vi "ThreadUI.vi"(4 "数据通知器":refnum<notifier>, 5 "Angle Data Queue":refnum<queue> caption="角度数据队列", 6 "User Event - Stop":refnum<user-event> caption="用户事件－停止", 7 "Analog Data Queue":refnum<queue> caption="模拟数据队列", 8 "error in (no error)":errorcluster caption="错误输入（无错误）", 10 "Measurement UI Controls":T1 caption="测量UI控件", 11 "Message Queues":T2 caption="消息队列") -> (0 "error out":errorcluster caption="错误输出")   [LabVIEW 2015]
uses:
  support/Message Queue/All Message Queues.ctl
  support/Message Queue/Message Cluster.ctl
  controls/UI Data.ctl
  Settings/Settings.ctl
  Acquisition/Hardware Configuration.ctl
  Logging/Logging Configuration.ctl
  Action/Hardware Configuration.ctl
  TaskMan/TaskMan Configuration.ctl
  TaskMan/TaskSettings.ctl
  controls/UI State.ctl
  Measure Type.ctl
  <vilib>/Analysis/baseanly.llb/Mean (DBL).vi
  support/Message Queue/Enqueue Message (Single).vi
  <vilib>/Utility/xml.llb/Write to XML File(string).vi
  <vilib>/Utility/error.llb/Error Cluster From Error Code.vi
  <vilib>/ErrorRing/Error Ring.xnode
  support/Message Queue/Message Queue.lvlib
  Acquisition/Acquisition.lvlib
  Logging/Logging.lvlib
  Action/Action.lvlib
  Settings/Settings.lvlib
  TaskMan/TaskMan.lvlib
  support/User Event - Stop/User Event - Stop.lvlib
  <vilib>/Analysis/NI_AALBase.lvlib
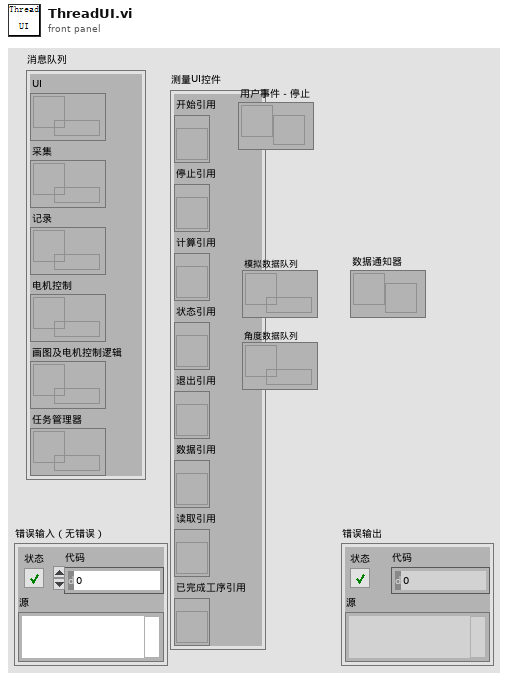
[diagram p1: front panel]
types:
  T1 = typedef "UI Data.ctl" = cluster{"Start Ref":refnum<vi>, "Stop Ref":refnum<vi>, "calculate Ref":refnum<vi>, "Status Ref":refnum<vi>, "Exit Ref":refnum<vi>, "read Ref":refnum<vi>, "clean Ref":refnum<vi>, "Finish Ref":refnum<vi>}
  T2 = typedef "Message Queue.lvlib/All Message Queues.ctl" = cluster{"UI":refnum<queue>, "Acquisition":refnum<queue>, "Logging":refnum<queue>, "plot logic":refnum<queue>, "Action Control":refnum<queue>, "TaskMan":refnum<queue>}
  T3 = typedef "UI State.ctl" = enum16{"Idle", "Acquiring and Logging", "Waiting for Exit", "Waiting for Exit (Acq Stopped)", "Waiting for Exit (Log Stopped)", "Waiting for Stop", "Waiting for Stop (Acq Stopped)", "Waiting for Stop (Log Stopped)"}
  T4 = typedef "Settings.lvlib/Settings.ctl" = cluster{"Hardware Configuration":T5, "Logging Configuration":T6, "Action Configuration":T7, "所有测试项目任务":T18}
  T5 = typedef "Acquisition.lvlib/Hardware Configuration.ctl" = cluster{"电压读取设置":cluster{"DAQmx Channel":tag, "Max Input":dbl, "Min Input":dbl, "Sample Rate":dbl, "Sample Number":i32, "DAQmx Task":refnum<k21>, "device in":tag}, "角度传感器设置":cluster{"counter":tag, "units":i32, "分辨率":i32, "初始角度":dbl, "DecodingType":i32, "A相端口":tag, "B相端口":tag, "task in":refnum<k21>}}
  T6 = typedef "Logging.lvlib/Logging Configuration.ctl" = cluster{"Log File Base Path":path, "电压传感器转换率":dbl[], "电压传感器本底":dbl[], "测试模式是否需要保存数据？":bool}
  T7 = typedef "Action.lvlib/Hardware Configuration.ctl" = cluster{"PLC设置":T8, "动作设置":T9, "电机设置":T13, "所有测试电机转动逻辑":T14}
  T8 = typedef "Action.lvlib/PLC设置.ctl" = cluster{"ActLogicalStationNumber":i32, "ActUtlType":refnum<k7>}
  T9 = typedef "Action.lvlib/动作设置.ctl" = cluster{"自动跳法测试动作":T10, "其他动作":T12}
  T10 = typedef "Action.lvlib/自动调阀测试动作设置.ctl" = cluster{"夹紧阀总":T11, "夹紧/松阀芯":T11, "方向机供油":T11, "扭杆紧/松":T11, "电机使能":T11, "内泄漏开":T11, "内泄漏停":T11, "数控钻孔启动":T11, "托起缸上":T11, "托起缸下":T11, "内泄漏放油":T11, "读取开始按钮":T11, "读取压销启动":T11, "读取压销完成":T11, "放松阀总":T11, "卡盘松紧":T11}
  T11 = typedef "Action.lvlib/PLC控制指令.ctl" = cluster{"变量类型":u32, "PLC地址":i32, "size":i32, "写入数据(写入时有效)":i16}
  T12 = typedef "Action.lvlib/其他动作设置 .ctl" = cluster{"其他指令1":T11, "其他指令2":T11, "其他指令3":T11, "其他指令4":T11, "其他指令5":T11}
  T13 = typedef "Action.lvlib/电机控制设置.ctl" = cluster{"counter":tag, "方向端口":tag, "当前方向":bool, "频率":dbl, "DAQmx Task":refnum<k21>, "一圈脉冲数":i32}
  T14 = typedef "Action.lvlib/所有测试电机转动逻辑.ctl" = cluster{"啮合测试电机转动逻辑":T15, "退回测试电机转动逻辑":T15, "功能测试电机转动逻辑":T15, "力特性测试电机转动逻辑":T15, "自动调阀测试分中电机转动逻辑":T15, "自动调阀测试对中电机转动逻辑":T15, "内泄漏电机转动逻辑":T15}
  T15 = typedef "Action.lvlib/电机转动逻辑1.ctl" = cluster{"反转判断条件1":T16, "停止判断条件1":T17}
  T16 = typedef "Action.lvlib/反转判断条件1.ctl" = cluster{"传感器序号":i32, "条件":enum16{"小于", "大于", "等于"}, "值":dbl, "条件判断时间间隔":i32}
  T17 = typedef "Action.lvlib/停止判断条件1.ctl" = cluster{"传感器序号":i32, "正转/反转":enum16{"正转", "反转"}, "反转次数":i32, "停止角度":dbl, "停止误差范围":dbl}
  T18 = typedef "TaskMan.lvlib/TaskMan Configuration.ctl" = cluster{"全自动调阀任务列表":T19}
  T19 = typedef "TaskMan.lvlib/全自动调阀任务列表.ctl" = T20[]
  T20 = typedef "TaskMan.lvlib/TaskSettings.ctl" = cluster{"任务指令":string, "等待时间":dbl}
  T21 = typedef "Measure Type.ctl" = enum16{"啮合", "退回", "功能", "力特性", "内泄漏", "分中", "对中"}
  T22 = enum8{"Enabled", "Disabled", "Disabled and Grayed Out"}
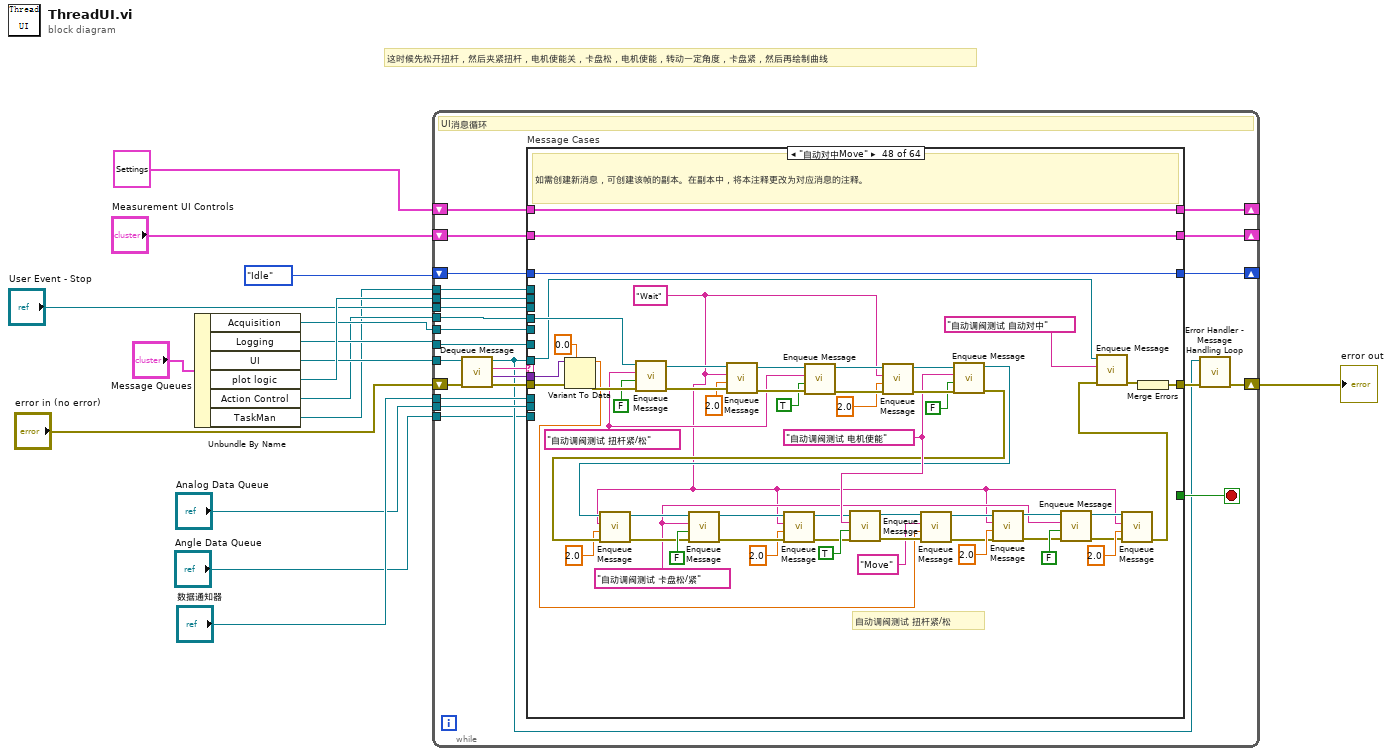
[diagram p0: block diagram]
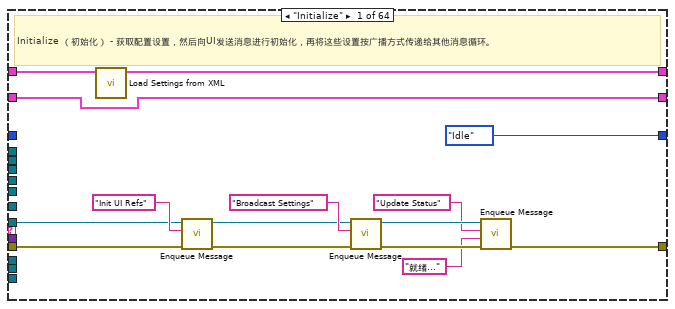
[diagram p2: hidden frame]
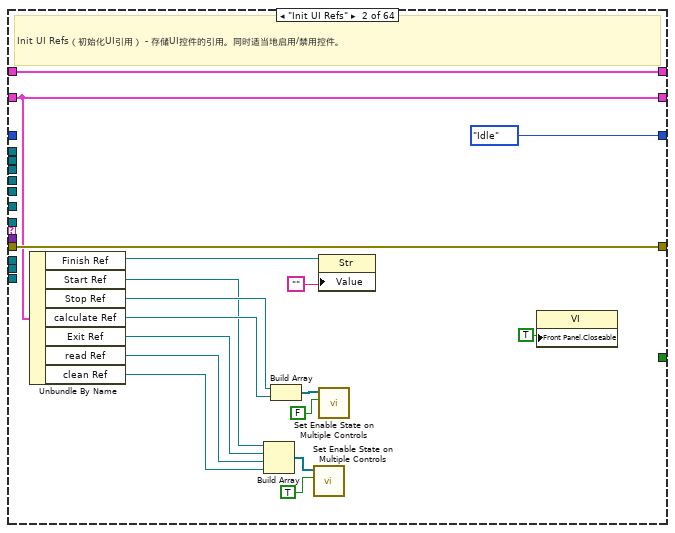
[diagram p3: hidden frame]
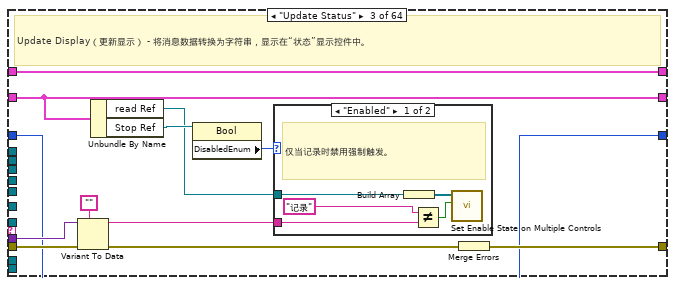
[diagram p4: hidden frame]
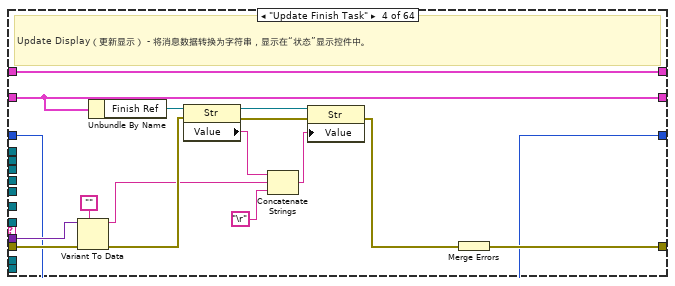
[diagram p6: hidden frame]
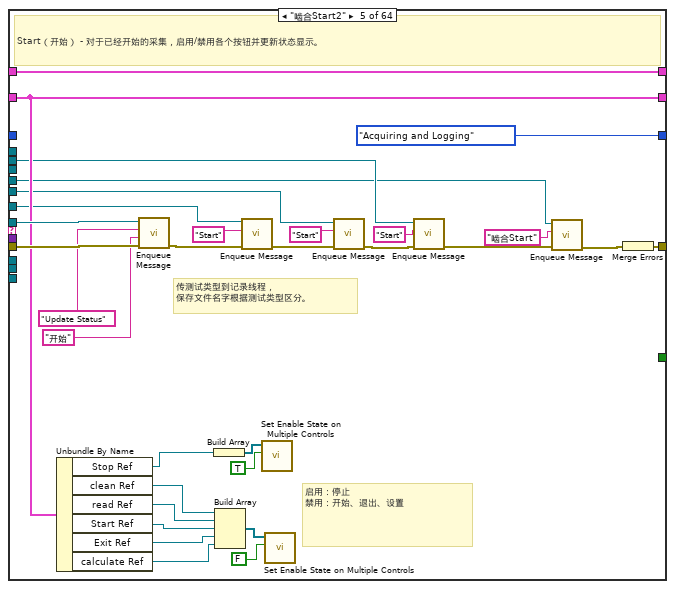
[diagram p7: hidden frame]
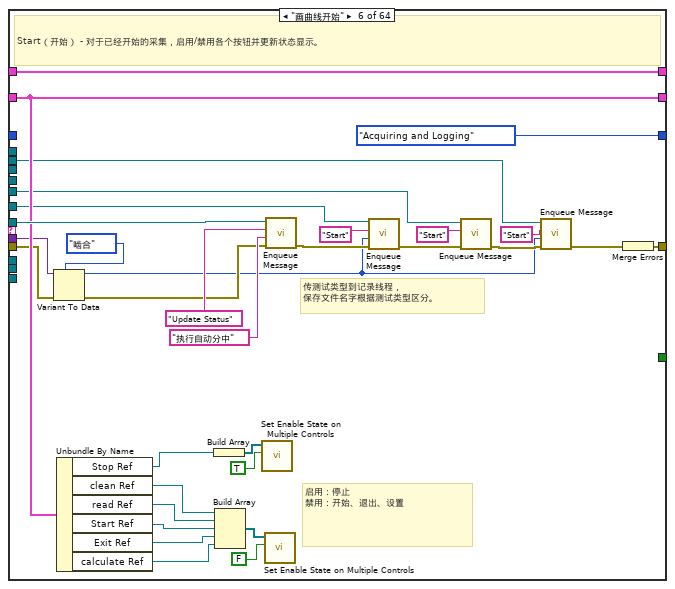
[diagram p8: hidden frame]
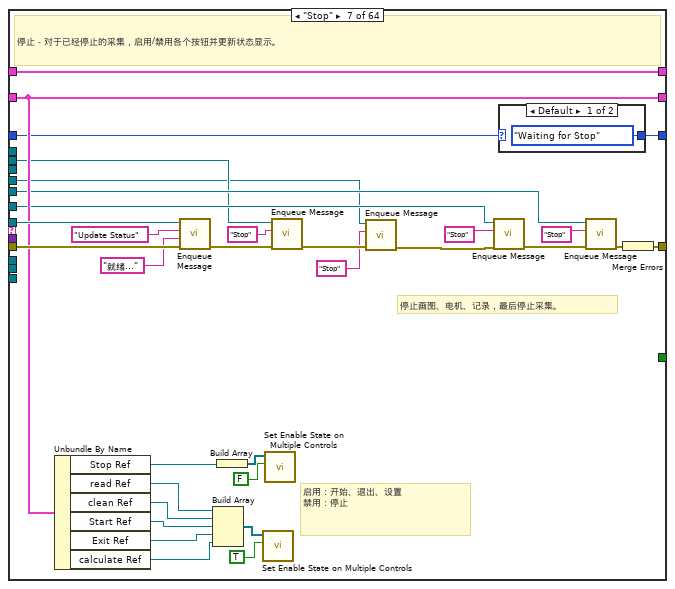
[diagram p9: hidden frame]
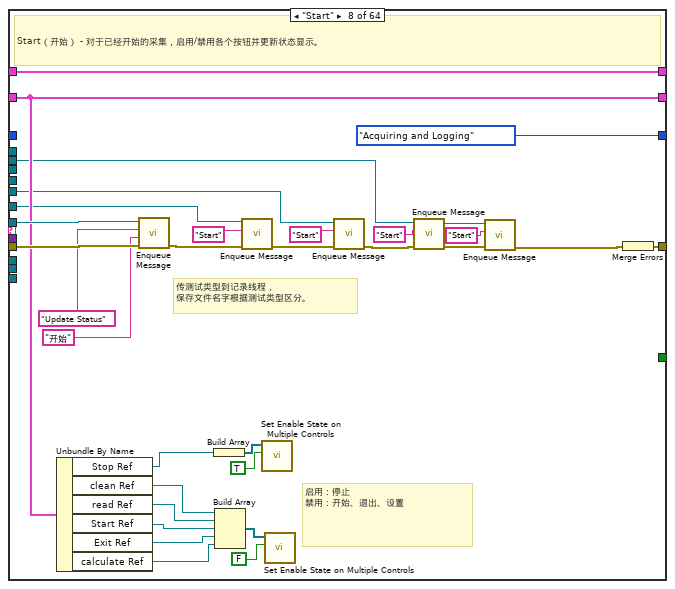
[diagram p11: hidden frame]
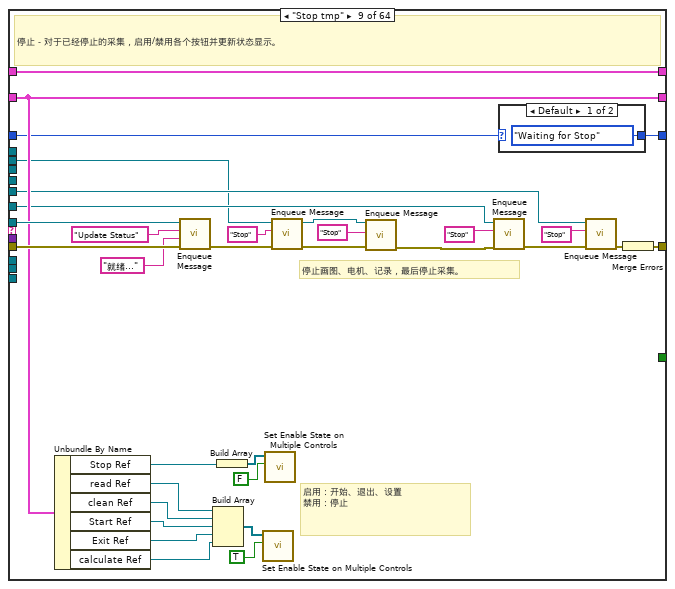
[diagram p12: hidden frame]
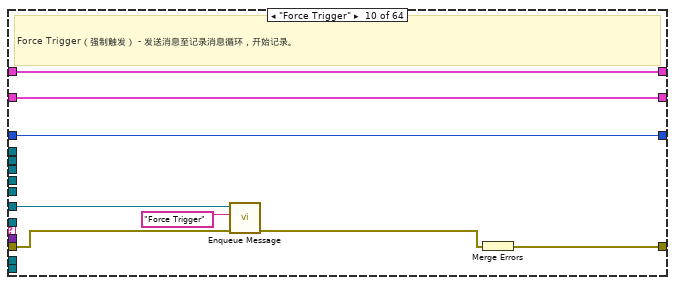
[diagram p14: hidden frame]
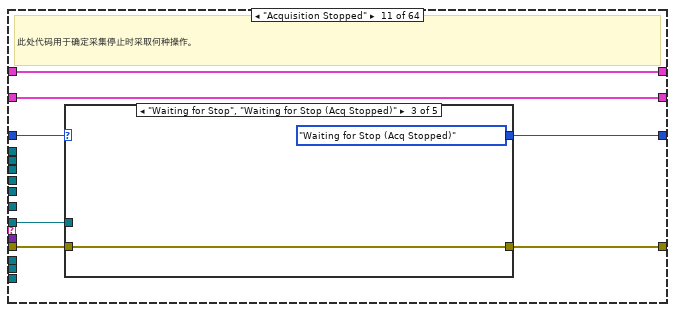
[diagram p15: hidden frame]
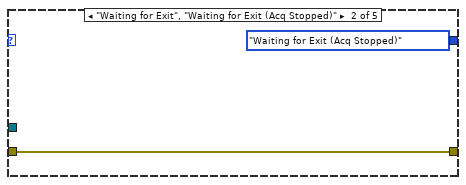
[diagram p17: hidden frame]
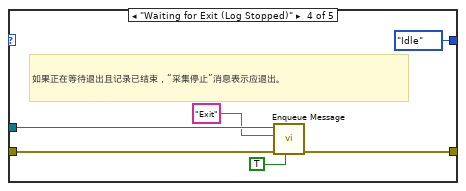
[diagram p18: hidden frame]
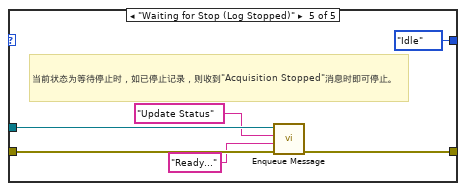
[diagram p19: hidden frame]
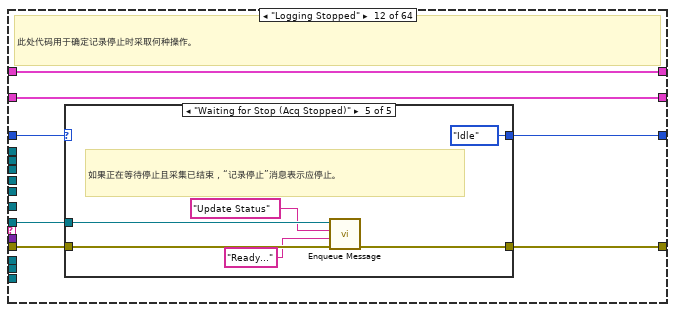
[diagram p20: hidden frame]
diagram:
  # "这时候先松开扭杆，然后夹紧扭杆，电机使能关，卡盘松，电机使能，转动一定角度，卡盘紧，然后再绘制曲线"
  n1 = Unbundle By Name("Message Queues") -> ("Acquisition"=w12:refnum<queue>, "Logging"=w13:refnum<queue>, "UI"=w14:refnum<queue>, "plot logic"=w15:refnum<queue>, "Action Control"=w2:refnum<queue>, "TaskMan"=w1:refnum<queue>)
  n2 = while {
    tunnel: w14 -> [w34]
    tunnel: "User Event - Stop" -> [w39]
    shift-right: [w24] -> w4
    shift-left: "error in (no error)" -> [w38]
    shift-right: [w33] -> _
    shift-left: T4 {"Hardware Configuration"={"电压读取设置"={"DAQmx Channel"="", "Max Input"=0.0, "Min Input"=0.0, "Sample Rate"=0.0, "Sample Number"=0, "DAQmx Task"="", "device in"=""}, "角度传感器设置"={"counter"="Dev1/ctr0", "units"=10146, "分辨率"=0, "初始角度"=0.0, "DecodingType"=10092, "A相端口"="/Dev1/PFI8", "B相端口"="/Dev1/PFI8", "task in"=""}}, "Logging Configuration"={"Log File Base Path"=path "", "电压传感器转换率"=[], "电压传感器本底"=[], "测试模式是否需要保存数据？"=FALSE}, "Action Configuration"={"PLC设置"={"ActLogicalStationNumber"=9600, "ActUtlType"=refnum}, "动作设置"={"自动跳法测试动作"={"夹紧阀总"={"变量类型"=2, "PLC地址"=0, "size"=0, "写入数据(写入时有效)"=0}, "夹紧/松阀芯"={"变量类型"=2, "PLC地址"=0, "size"=0, "写入数据(写入时有效)"=0}, "方向机供油"={"变量类型"=2, "PLC地址"=0, "size"=0, "写入数据(写入时有效)"=0}, "扭杆紧/松"={"变量类型"=2, "PLC地址"=0, "size"=0, "写入数据(写入时有效)"=0}, "电机使能"={"变量类型"=2, "PLC地址"=0, "size"=0, "写入数据(写入时有效)"=0}, "内泄漏开"={"变量类型"=2, "PLC地址"=0, "size"=0, "写入数据(写入时有效)"=0}, "内泄漏停"={"变量类型"=2, "PLC地址"=0, "size"=0, "写入数据(写入时有效)"=0}, "数控钻孔启动"={"变量类型"=2, "PLC地址"=0, "size"=0, "写入数据(写入时有效)"=0}, "托起缸上"={"变量类型"=2, "PLC地址"=0, "size"=0, "写入数据(写入时有效)"=0}, "托起缸下"={"变量类型"=2, "PLC地址"=0, "size"=0, "写入数据(写入时有效)"=0}, "内泄漏放油"={"变量类型"=2, "PLC地址"=0, "size"=0, "写入数据(写入时有效)"=0}, "读取开始按钮"={"变量类型"=2, "PLC地址"=0, "size"=0, "写入数据(写入时有效)"=0}, "读取压销启动"={"变量类型"=2, "PLC地址"=0, "size"=0, "写入数据(写入时有效)"=0}, "读取压销完成"={"变量类型"=2, "PLC地址"=0, "size"=0, "写入数据(写入时有效)"=0}, "放松阀总"={"变量类型"=2, "PLC地址"=0, "size"=0, "写入数据(写入时有效)"=0}, "卡盘松紧"={"变量类型"=2, "PLC地址"=0, "size"=0, "写入数据(写入时有效)"=0}}, "其他动作"={"其他指令1"={"变量类型"=2, "PLC地址"=0, "size"=0, "写入数据(写入时有效)"=0}, "其他指令2"={"变量类型"=2, "PLC地址"=0, "size"=0, "写入数据(写入时有效)"=0}, "其他指令3"={"变量类型"=2, "PLC地址"=0, "size"=0, "写入数据(写入时有效)"=0}, "其他指令4"={"变量类型"=2, "PLC地址"=0, "size"=0, "写入数据(写入时有效)"=0}, "其他指令5"={"变量类型"=2, "PLC地址"=0, "size"=0, "写入数据(写入时有效)"=0}}}, "电机设置"={"counter"="Dev1/ctr0", "方向端口"="", "当前方向"=FALSE, "频率"=0.0, "DAQmx Task"="", "一圈脉冲数"=0}, "所有测试电机转动逻辑"={"啮合测试电机转动逻辑"={"反转判断条件1"={"传感器序号"=0, "条件"=enum."小于", "值"=0.0, "条件判断时间间隔"=0}, "停止判断条件1"={"传感器序号"=0, "正转/反转"=enum."正转", "反转次数"=0, "停止角度"=0.0, "停止误差范围"=0.0}}, "退回测试电机转动逻辑"={"反转判断条件1"={"传感器序号"=0, "条件"=enum."小于", "值"=0.0, "条件判断时间间隔"=0}, "停止判断条件1"={"传感器序号"=0, "正转/反转"=enum."正转", "反转次数"=0, "停止角度"=0.0, "停止误差范围"=0.0}}, "功能测试电机转动逻辑"={"反转判断条件1"={"传感器序号"=0, "条件"=enum."小于", "值"=0.0, "条件判断时间间隔"=0}, "停止判断条件1"={"传感器序号"=0, "正转/反转"=enum."正转", "反转次数"=0, "停止角度"=0.0, "停止误差范围"=0.0}}, "力特性测试电机转动逻辑"={"反转判断条件1"={"传感器序号"=0, "条件"=enum."小于", "值"=0.0, "条件判断时间间隔"=0}, "停止判断条件1"={"传感器序号"=0, "正转/反转"=enum."正转", "反转次数"=0, "停止角度"=0.0, "停止误差范围"=0.0}}, "自动调阀测试分中电机转动逻辑"={"反转判断条件1"={"传感器序号"=0, "条件"=enum."小于", "值"=0.0, "条件判断时间间隔"=0}, "停止判断条件1"={"传感器序号"=0, "正转/反转"=enum."正转", "反转次数"=0, "停止角度"=0.0, "停止误差范围"=0.0}}, "自动调阀测试对中电机转动逻辑"={"反转判断条件1"={"传感器序号"=0, "条件"=enum."小于", "值"=0.0, "条件判断时间间隔"=0}, "停止判断条件1"={"传感器序号"=0, "正转/反转"=enum."正转", "反转次数"=0, "停止角度"=0.0, "停止误差范围"=0.0}}, "内泄漏电机转动逻辑"={"反转判断条件1"={"传感器序号"=0, "条件"=enum."小于", "值"=0.0, "条件判断时间间隔"=0}, "停止判断条件1"={"传感器序号"=0, "正转/反转"=enum."正转", "反转次数"=0, "停止角度"=0.0, "停止误差范围"=0.0}}}}, "所有测试项目任务"={"全自动调阀任务列表"=[]}} ("Settings") -> [w32]
    shift-right: [w30] -> _
    shift-left: "Measurement UI Controls" -> [w31]
    tunnel: w12 -> [w29]
    tunnel: w13 -> [w28]
    tunnel: "数据通知器" -> [w27]
    tunnel: "Analog Data Queue" -> [w26]
    shift-right: [w21] -> _
    shift-left: UI_State."Idle" ("UI State") -> [w22]
    tunnel: w15 -> [w19]
    tunnel: "Angle Data Queue" -> [w20]
    tunnel: w2 -> [w18]
    tunnel: w1 -> [w17]
    stop <- w40 stop-if-true
    # "UI消息循环"
    n3 = call "Dequeue Message.vi"("error in (no error)"=w38, "Message Queue"=w34) -> ("error out"=w37:errorcluster, "Message Data"=w35:variant, "Message"=w36:string, "dup Message Queue"=w23:refnum<queue>)  [unwired: 6 in]
    n4 = case "Message Cases" shown="\"自动对中Move\"" w36 {
      selector: w36 -> [_ _ _ _ _ _ _ _ _ _ _ _ _ _ _ _ _ _ _ _ _ _ _ _ _ _ _ _ _ _ _ _ _ _ _ _ _ _ _ _ _ _ _ _ _ _ _ _ _ _ _ _ _ _ _ _ _ _ _ _ _ _ _ w946]
      tunnel: w23 -> [w45 _ _ _ w135 w167 w199 w232 w264 _ w276 w301 _ w350 w370 w376 w415 _ _ _ _ w475 w487 w499 w511 _ _ w537 _ _ _ _ _ _ _ w621 _ _ _ _ _ w686 _ _ w712 _ _ w740 w797 _ _ _ _ _ _ _ _ w880 w901 _ _ _ w934 _]
      tunnel: w37 -> [w44 w72 w83 w104 w134 w141 w198 w231 w263 w272 w278 w303 w333 w351 w363 w375 w422 w429 w436 w447 w460 w474 w486 w498 w510 w516 w526 w540 w552 w566 w574 w585 w594 w603 w612 w619 w636 w645 w653 w662 w671 w685 w694 w700 w710 w727 w735 w790 w799 w811 w819 w828 w836 w844 w853 w862 w871 w878 w900 w907 w916 w925 w932 _]
      tunnel: [w51 w72 w84 w105 w136 w168 w200 w233 w265 w275 w277 w302 w343 w348 w366 w374 w423 w428 w443 w452 w464 w476 w488 w500 w512 w519 w530 w543 w556 w569 w581 w589 w598 w607 w616 w631 w640 w649 w657 w666 w675 w687 w699 w707 w722 w731 w739 w794 w806 w815 w823 w832 w840 w848 w857 w866 w875 w890 w902 w911 w920 w929 w944 w947] -> w25
      tunnel: [_ _ _ _ _ _ _ _ _ _ _ _ _ _ _ _ TRUE _ _ _ _ _ _ _ _ _ _ _ _ _ _ _ _ _ _ _ _ _ _ _ _ _ _ _ _ _ _ _ _ _ _ _ _ _ _ _ _ _ _ _ _ _ _ _] -> w40
      tunnel: w35 -> [_ _ w82 w103 _ w140 _ _ _ _ _ _ _ _ w362 _ _ _ w434 w444 w459 _ _ _ _ _ _ _ _ _ w572 _ w590 w599 w608 _ w632 w641 _ w658 w667 _ w693 _ _ _ _ w789 _ w807 _ w824 _ _ _ _ _ _ _ _ _ _ _ _]
      tunnel: w39 -> [_ _ _ _ _ _ _ _ _ _ _ _ _ _ _ _ w421 _ _ _ _ _ _ _ _ _ _ _ _ _ _ _ _ _ _ _ _ _ _ _ _ _ _ _ _ _ _ _ _ _ _ _ _ _ _ _ _ _ _ _ _ _ _ _]
      tunnel: [w54 w71 w79 w101 w133 w166 w197 w230 w262 w274 w282 w307 w341 w349 w372 w379 w419 w427 w430 w451 w463 w473 w485 w497 w509 w514 w527 w533 w553 w564 w580 w588 w595 w604 w613 w630 w637 w646 w654 w663 w672 w684 w688 w702 w721 w728 w736 w793 w803 w812 w820 w829 w837 w847 w856 w865 w874 w889 w899 w910 w919 w928 w943 w949] -> w33
      tunnel: w32 -> [w55 w71 w79 w101 w133 w166 w197 w230 w262 w274 w282 w307 w341 w352 w372 w379 w419 w427 w432 w451 w463 w473 w485 w497 w509 w514 w527 w534 w553 w564 w580 w588 w595 w604 w613 w630 w637 w646 w654 w663 w672 w684 w688 w702 w721 w728 w736 w793 w803 w812 w820 w829 w837 w847 w856 w865 w874 w889 w899 w910 w919 w928 w943 w949]
      tunnel: w31 -> [w47 w58 w78 w100 w130 w163 w194 w227 w259 w273 w281 w306 w338 w347 w371 w378 w418 w426 w442 w450 w462 w471 w483 w495 w507 w518 w529 w542 w555 w568 w579 w587 w597 w606 w615 w628 w639 w648 w656 w665 w674 w682 w698 w706 w719 w730 w738 w792 w805 w814 w822 w831 w839 w846 w855 w864 w873 w887 w897 w909 w918 w927 w941 w948]
      tunnel: [w47 w58 w78 w100 w130 w163 w194 w227 w259 w273 w281 w306 w338 w347 w371 w378 w418 w426 w442 w450 w462 w471 w483 w495 w507 w518 w529 w542 w555 w568 w579 w587 w597 w606 w615 w628 w639 w648 w656 w665 w674 w682 w698 w706 w719 w730 w738 w792 w805 w814 w822 w831 w839 w846 w855 w864 w873 w887 w897 w909 w918 w927 w941 w948] -> w30
      tunnel: w29 -> [_ _ _ _ w118 w151 w182 w215 w247 _ _ _ w337 _ _ _ w417 _ _ _ _ _ _ _ _ _ w525 _ w551 _ _ _ _ _ _ _ _ _ _ _ _ _ _ _ _ _ _ _ _ _ _ _ _ _ _ _ _ _ _ _ _ _ _ _]
      tunnel: w28 -> [_ _ _ _ w120 w153 w185 w217 w250 w269 _ _ w336 _ _ _ w416 _ _ _ _ _ _ _ _ _ w522 _ w548 _ w576 w582 _ _ _ _ _ _ _ _ _ _ _ w701 _ w723 w732 _ _ _ _ _ _ _ _ _ _ _ _ _ _ _ _ _]
      tunnel: w27 -> [_ _ _ _ _ _ _ _ _ _ _ _ _ _ _ _ w414 _ _ _ _ _ _ _ _ _ _ _ _ _ _ _ _ _ _ _ _ _ _ _ _ _ _ _ _ _ _ _ _ _ _ _ _ _ _ _ _ _ _ _ _ _ _ _]
      tunnel: w26 -> [_ _ _ _ _ _ _ _ _ _ _ _ _ _ _ _ w411 _ _ _ _ _ _ _ _ _ _ _ _ _ _ _ _ _ _ _ _ _ _ _ _ _ _ _ _ _ _ _ _ _ _ _ _ _ _ _ _ _ _ _ _ _ _ _]
      tunnel: w22 -> [_ _ w73 w99 _ _ w180 _ w245 w268 w280 w305 w335 w346 w365 w377 _ w425 w441 w449 w461 w466 w478 w490 w502 w517 w528 w541 w554 w567 w578 w586 w596 w605 w614 w623 w638 w647 w655 w664 w673 w677 w697 w705 w714 w729 w737 w791 w804 w813 w821 w830 w838 w845 w854 w863 w872 w882 w892 w908 w917 w926 w936 w945]
      tunnel: [UI_State."Idle" ("UI State") UI_State."Idle" ("UI State") w73 w99 UI_State."Acquiring and Logging" ("UI State") UI_State."Acquiring and Logging" ("UI State") w179 UI_State."Acquiring and Logging" ("UI State") w244 w268 w279 w304 w335 w346 w365 w373 UI_State."Idle" ("UI State") w425 w441 w449 w461 w466 w478 w490 w502 w517 w528 w541 w554 w567 w578 w586 w596 w605 w614 w623 w638 w647 w655 w664 w673 w677 w697 w705 w714 w729 w737 w791 w804 w813 w821 w830 w838 w845 w854 w863 w872 w882 w892 w908 w917 w926 w936 w945] -> w21
      tunnel: w20 -> [_ _ _ _ _ _ _ _ _ _ _ _ _ _ _ _ w406 _ _ _ _ _ _ _ _ _ _ _ _ _ _ _ _ _ _ _ _ _ _ _ _ _ _ _ _ _ _ _ _ _ _ _ _ _ _ _ _ _ _ _ _ _ _ _]
      tunnel: w19 -> [_ _ _ _ w112 w145 w172 w209 w237 _ _ _ _ _ _ _ w405 _ _ w445 _ _ _ _ _ _ _ _ _ w559 _ _ _ _ _ _ _ _ _ _ _ _ _ _ _ _ _ _ _ _ _ _ _ _ _ _ _ _ _ _ _ _ _ _]
      tunnel: w18 -> [_ _ _ _ w106 _ w169 _ _ _ _ _ w332 _ _ _ w404 _ _ _ w456 w468 w480 w492 w504 _ _ _ _ _ _ _ w592 w601 w610 w625 w634 w643 w651 w660 w669 w679 w696 _ w716 _ _ w785 _ w809 w817 w826 w834 _ w850 w859 w868 w884 w894 w904 w913 w922 w938 _]
      tunnel: w17 -> [_ _ _ _ _ _ _ _ _ _ _ _ w328 _ _ _ w403 _ _ _ _ _ _ _ _ _ _ _ _ _ _ _ _ _ _ _ _ _ _ _ _ _ _ _ _ _ _ _ w800 _ _ _ _ w842 _ _ _ _ _ _ _ _ _ _]
      frame "Initialize" {
        # "Initialize （初始化） - 获取配置设置，然后向UI发送消息进行初始化，再将这些设置按广播方式传递给其他消息循环。"
        n5 = call "Load Settings from XML.vi"("Settings in"=w55) -> ("Settings out"=w54:T4)  [unwired: 9 in, 1 out]
        n6 = call-poly "Enqueue Message.vi"("error in (no error)"=w44, "Message"="Init UI Refs", "Message Queue"=w45) -> ("error out"=w42:errorcluster, "dup Message Queue"=w43:refnum<queue>)  [unwired: 7 in]
        n7 = call-poly "Enqueue Message.vi"("error in (no error)"=w42, "Message"="Broadcast Settings", "Message Queue"=w43) -> ("error out"=w53:errorcluster, "dup Message Queue"=w52:refnum<queue>)  [unwired: 7 in]
        n8 = call-poly "Enqueue Message.vi"("error in (no error)"=w53, "Message Data"="就绪..." ("Ready..."), "Message"="Update Status", "Message Queue"=w52) -> ("error out"=w51:errorcluster)  [unwired: 6 in, 1 out]
      }
      frame "Init UI Refs" {
        # "Init UI Refs（初始化UI引用） - 存储UI控件的引用。同时适当地启用/禁用控件。"
        n9 = Unbundle By Name(w58) -> ("Finish Ref"=w57:refnum<vi>, "Start Ref"=w62:refnum<vi>, "Stop Ref"=w64:refnum<vi>, "calculate Ref"=w63:refnum<vi>, "Exit Ref"=w61:refnum<vi>, "read Ref"=w60:refnum<vi>, "clean Ref"=w59:refnum<vi>)
        n10 = Build Array(w62, w61, w60, w59) -> (w68:refnum<vi>[])
        n11 = Build Array(w64, w63) -> (w66:refnum<vi>[])
        n12 = call "Set Enable State on Multiple Controls.vi"("Enable?"=TRUE, "Controls"=w68) -> ()  [unwired: 10 in]
        n13 = property class="Str"(reference=w57, "Value"="") -> ()  [unwired: 1 in, 2 out]
        n14 = call "Set Enable State on Multiple Controls.vi"("Enable?"=FALSE, "Controls"=w66) -> ()  [unwired: 10 in]
        n15 = property class="VI"("Front Panel.Closeable"=TRUE ("Front Panel Window:Closeable")) -> ()  [unwired: 2 in, 2 out]
      }
      frame "Update Status" {
        # "Update Display（更新显示） - 将消息数据转换为字符串，显示在“状态”显示控件中。"
        n16 = Variant To Data(error in=w83, type="", Variant=w82) -> (data=w75:string, error out=w80:errorcluster)
        n17 = Unbundle By Name(w78) -> ("read Ref"=w74:refnum<vi>, "Stop Ref"=w77:refnum<vi>)
        n18 = property class="Bool"(reference=w77) -> ("DisabledEnum"=w76:T22)  [unwired: 1 in, 2 out]
        n19 = case shown="\"Enabled\"" w76 {
          tunnel: w75 -> [w87 _]
          tunnel: w74 -> [w88 _]
          frame "Enabled" {
            # "仅当记录时禁用强制触发。"
            n20 = Build Array(w88) -> (w89:refnum<vi>[])
            n21 = Not Equal?(x="记录" ("Logging"), y=w87) -> (x != y?=w85:bool)
            n22 = call "Set Enable State on Multiple Controls.vi"("Enable?"=w85, "Controls"=w89) -> ()  [unwired: 10 in]
          }
          frame "Disabled", Default {
          }
        }
        n23 = Merge Errors(w80) -> (w84:errorcluster)
      }
      frame "Update Finish Task" {
        # "Update Display（更新显示） - 将消息数据转换为字符串，显示在“状态”显示控件中。"
        n24 = Variant To Data(error in=w104, type="", Variant=w103) -> (data=w91:string, error out=w94:errorcluster)
        n25 = Unbundle By Name(w100) -> ("Finish Ref"=w98:refnum<vi>)
        n26 = property class="Str"(reference=w98, error in=w94) -> (reference out=w96:refnum<vi>, error out=w95:errorcluster, "Value"=w97:string)
        n27 = Concatenate Strings(w97, w91, "\r") -> (w93:string)
        n28 = property class="Str"(reference=w96, error in=w95, "Value"=w93) -> (error out=w92:errorcluster)  [unwired: 1 out]
        n29 = Merge Errors(w92) -> (w105:errorcluster)
      }
      frame "啮合Start2" {
        # "传测试类型到记录线程，\n保存文件名字根据测试类型区分。"
        # "启用：停止\n禁用：开始、退出、设置"
        # "Start（开始） - 对于已经开始的采集，启用/禁用各个按钮并更新状态显示。"
        n30 = Unbundle By Name(w130) -> ("Stop Ref"=w113:refnum<vi>, "clean Ref"=w114:refnum<vi>, "read Ref"=w115:refnum<vi>, "Start Ref"=w125:refnum<vi>, "Exit Ref"=w124:refnum<vi>, "calculate Ref"=w123:refnum<vi>)
        n31 = call-poly "Enqueue Message.vi"("error in (no error)"=w134, "Message Data"="开始" ("Waiting for trigger"), "Message"="Update Status", "Message Queue"=w135) -> ("error out"=w122:errorcluster)  [unwired: 6 in, 1 out]
        n32 = Build Array(w113) -> (w127:refnum<vi>[])
        n33 = Build Array(w114, w115, w125, w124, w123) -> (w128:refnum<vi>[])
        n34 = call-poly "Enqueue Message.vi"("error in (no error)"=w122, "Message"="Start", "Message Queue"=w120) -> ("error out"=w119:errorcluster)  [unwired: 7 in, 1 out]
        n35 = call "Set Enable State on Multiple Controls.vi"("Enable?"=TRUE, "Controls"=w127) -> ()  [unwired: 10 in]
        n36 = call "Set Enable State on Multiple Controls.vi"("Enable?"=FALSE, "Controls"=w128) -> ()  [unwired: 10 in]
        n37 = call-poly "Enqueue Message.vi"("error in (no error)"=w119, "Message"="Start", "Message Queue"=w118) -> ("error out"=w110:errorcluster)  [unwired: 7 in, 1 out]
        n38 = call-poly "Enqueue Message.vi"("error in (no error)"=w110, "Message"="Start", "Message Queue"=w112) -> ("error out"=w109:errorcluster)  [unwired: 7 in, 1 out]
        n39 = call-poly "Enqueue Message.vi"("error in (no error)"=w109, "Message"="啮合Start", "Message Queue"=w106) -> ("error out"=w107:errorcluster)  [unwired: 7 in, 1 out]
        n40 = Merge Errors(w107) -> (w136:errorcluster)
      }
      frame "画曲线开始" {
        # "传测试类型到记录线程，\n保存文件名字根据测试类型区分。"
        # "启用：停止\n禁用：开始、退出、设置"
        # "Start（开始） - 对于已经开始的采集，启用/禁用各个按钮并更新状态显示。"
        n41 = Variant To Data(error in=w141, type=Measure_Type."啮合" ("测试类型"), Variant=w140) -> (data=w137:T21, error out=w139:errorcluster)
        n42 = Unbundle By Name(w163) -> ("Stop Ref"=w146:refnum<vi>, "clean Ref"=w147:refnum<vi>, "read Ref"=w148:refnum<vi>, "Start Ref"=w158:refnum<vi>, "Exit Ref"=w157:refnum<vi>, "calculate Ref"=w156:refnum<vi>)
        n43 = Build Array(w146) -> (w160:refnum<vi>[])
        n44 = Build Array(w147, w148, w158, w157, w156) -> (w161:refnum<vi>[])
        n45 = call "Set Enable State on Multiple Controls.vi"("Enable?"=TRUE, "Controls"=w160) -> ()  [unwired: 10 in]
        n46 = call "Set Enable State on Multiple Controls.vi"("Enable?"=FALSE, "Controls"=w161) -> ()  [unwired: 10 in]
        n47 = call-poly "Enqueue Message.vi"("error in (no error)"=w139, "Message Data"="执行自动分中" ("Waiting for trigger"), "Message"="Update Status", "Message Queue"=w167) -> ("error out"=w155:errorcluster)  [unwired: 6 in, 1 out]
        n48 = call-poly "Enqueue Message.vi"("error in (no error)"=w155, "Message Data"=w137, "Message"="Start", "Message Queue"=w153) -> ("error out"=w152:errorcluster)  [unwired: 6 in, 1 out]
        n49 = call-poly "Enqueue Message.vi"("error in (no error)"=w152, "Message"="Start", "Message Queue"=w151) -> ("error out"=w143:errorcluster)  [unwired: 7 in, 1 out]
        n50 = call-poly "Enqueue Message.vi"("error in (no error)"=w143, "Message Data"=w137, "Message"="Start", "Message Queue"=w145) -> ("error out"=w142:errorcluster)  [unwired: 6 in, 1 out]
        n51 = Merge Errors(w142) -> (w168:errorcluster)
      }
      frame "Stop" {
        # "停止画图、电机、记录，最后停止采集。"
        # "启用：开始、退出、设置\n禁用：停止"
        # "停止－对于已经停止的采集，启用/禁用各个按钮并更新状态显示。"
        n52 = Unbundle By Name(w194) -> ("Stop Ref"=w176:refnum<vi>, "read Ref"=w177:refnum<vi>, "clean Ref"=w178:refnum<vi>, "Start Ref"=w189:refnum<vi>, "Exit Ref"=w188:refnum<vi>, "calculate Ref"=w187:refnum<vi>)
        n53 = call-poly "Enqueue Message.vi"("error in (no error)"=w198, "Message Data"="就绪..." ("Ready..."), "Message"="Update Status", "Message Queue"=w199) -> ("error out"=w175:errorcluster)  [unwired: 6 in, 1 out]
        n54 = Build Array(w177, w178, w189, w188, w187) -> (w192:refnum<vi>[])
        n55 = Build Array(w176) -> (w191:refnum<vi>[])
        n56 = call "Set Enable State on Multiple Controls.vi"("Enable?"=TRUE, "Controls"=w192) -> ()  [unwired: 10 in]
        n57 = call "Set Enable State on Multiple Controls.vi"("Enable?"=FALSE, "Controls"=w191) -> ()  [unwired: 10 in]
        n58 = call-poly "Enqueue Message.vi"("error in (no error)"=w175, "Message"="Stop", "Message Queue"=w172) -> ("error out"=w174:errorcluster)  [unwired: 7 in, 1 out]
        n59 = call-poly "Enqueue Message.vi"("error in (no error)"=w174, "Message"="Stop", "Message Queue"=w169) -> ("error out"=w173:errorcluster)  [unwired: 7 in, 1 out]
        n60 = call-poly "Enqueue Message.vi"("error in (no error)"=w173, "Message"="Stop", "Message Queue"=w185) -> ("error out"=w184:errorcluster)  [unwired: 7 in, 1 out]
        n61 = case shown="Default" w180 {
          selector: w180 -> [_ w202]
          tunnel: [UI_State."Waiting for Stop" ("UI State") w202] -> w179
          frame Default {
          }
          frame "Waiting for Exit" {
          }
        }
        n62 = call-poly "Enqueue Message.vi"("error in (no error)"=w184, "Message"="Stop", "Message Queue"=w182) -> ("error out"=w183:errorcluster)  [unwired: 7 in, 1 out]
        n63 = Merge Errors(w183) -> (w200:errorcluster)
      }
      frame "Start" {
        # "传测试类型到记录线程，\n保存文件名字根据测试类型区分。"
        # "启用：停止\n禁用：开始、退出、设置"
        # "Start（开始） - 对于已经开始的采集，启用/禁用各个按钮并更新状态显示。"
        n64 = Unbundle By Name(w227) -> ("Stop Ref"=w210:refnum<vi>, "clean Ref"=w211:refnum<vi>, "read Ref"=w212:refnum<vi>, "Start Ref"=w222:refnum<vi>, "Exit Ref"=w221:refnum<vi>, "calculate Ref"=w220:refnum<vi>)
        n65 = call-poly "Enqueue Message.vi"("error in (no error)"=w231, "Message Data"="开始" ("Waiting for trigger"), "Message"="Update Status", "Message Queue"=w232) -> ("error out"=w219:errorcluster)  [unwired: 6 in, 1 out]
        n66 = Build Array(w210) -> (w224:refnum<vi>[])
        n67 = Build Array(w211, w212, w222, w221, w220) -> (w225:refnum<vi>[])
        n68 = call-poly "Enqueue Message.vi"("error in (no error)"=w219, "Message"="Start", "Message Queue"=w217) -> ("error out"=w216:errorcluster)  [unwired: 7 in, 1 out]
        n69 = call "Set Enable State on Multiple Controls.vi"("Enable?"=TRUE, "Controls"=w224) -> ()  [unwired: 10 in]
        n70 = call "Set Enable State on Multiple Controls.vi"("Enable?"=FALSE, "Controls"=w225) -> ()  [unwired: 10 in]
        n71 = call-poly "Enqueue Message.vi"("error in (no error)"=w216, "Message"="Start", "Message Queue"=w215) -> ("error out"=w207:errorcluster)  [unwired: 7 in, 1 out]
        n72 = call-poly "Enqueue Message.vi"("error in (no error)"=w207, "Message"="Start", "Message Queue"=w209) -> ("error out"=w206:errorcluster, "dup Message Queue"=w203:refnum<queue>)  [unwired: 7 in]
        n73 = call-poly "Enqueue Message.vi"("error in (no error)"=w206, "Message"="Start", "Message Queue"=w203) -> ("error out"=w204:errorcluster)  [unwired: 7 in, 1 out]
        n74 = Merge Errors(w204) -> (w233:errorcluster)
      }
      frame "Stop tmp" {
        # "停止画图、电机、记录，最后停止采集。"
        # "启用：开始、退出、设置\n禁用：停止"
        # "停止－对于已经停止的采集，启用/禁用各个按钮并更新状态显示。"
        n75 = Unbundle By Name(w259) -> ("Stop Ref"=w241:refnum<vi>, "read Ref"=w242:refnum<vi>, "clean Ref"=w243:refnum<vi>, "Start Ref"=w254:refnum<vi>, "Exit Ref"=w253:refnum<vi>, "calculate Ref"=w252:refnum<vi>)
        n76 = call-poly "Enqueue Message.vi"("error in (no error)"=w263, "Message Data"="就绪..." ("Ready..."), "Message"="Update Status", "Message Queue"=w264) -> ("error out"=w240:errorcluster)  [unwired: 6 in, 1 out]
        n77 = Build Array(w242, w243, w254, w253, w252) -> (w257:refnum<vi>[])
        n78 = Build Array(w241) -> (w256:refnum<vi>[])
        n79 = call "Set Enable State on Multiple Controls.vi"("Enable?"=TRUE, "Controls"=w257) -> ()  [unwired: 10 in]
        n80 = call "Set Enable State on Multiple Controls.vi"("Enable?"=FALSE, "Controls"=w256) -> ()  [unwired: 10 in]
        n81 = call-poly "Enqueue Message.vi"("error in (no error)"=w240, "Message"="Stop", "Message Queue"=w237) -> ("error out"=w239:errorcluster, "dup Message Queue"=w234:refnum<queue>)  [unwired: 7 in]
        n82 = call-poly "Enqueue Message.vi"("error in (no error)"=w239, "Message"="Stop", "Message Queue"=w234) -> ("error out"=w238:errorcluster)  [unwired: 7 in, 1 out]
        n83 = call-poly "Enqueue Message.vi"("error in (no error)"=w238, "Message"="Stop", "Message Queue"=w250) -> ("error out"=w249:errorcluster)  [unwired: 7 in, 1 out]
        n84 = case shown="Default" w245 {
          selector: w245 -> [_ w267]
          tunnel: [UI_State."Waiting for Stop" ("UI State") w267] -> w244
          frame Default {
          }
          frame "Waiting for Exit" {
          }
        }
        n85 = call-poly "Enqueue Message.vi"("error in (no error)"=w249, "Message"="Stop", "Message Queue"=w247) -> ("error out"=w248:errorcluster)  [unwired: 7 in, 1 out]
        n86 = Merge Errors(w248) -> (w265:errorcluster)
      }
      frame "Force Trigger" {
        # "Force Trigger（强制触发） - 发送消息至记录消息循环，开始记录。"
        n87 = call-poly "Enqueue Message.vi"("error in (no error)"=w272, "Message"="Force Trigger", "Message Queue"=w269) -> ("error out"=w271:errorcluster)  [unwired: 7 in, 1 out]
        n88 = Merge Errors(w271) -> (w275:errorcluster)
      }
      frame "Acquisition Stopped" {
        # "此处代码用于确定采集停止时采取何种操作。"
        n89 = case shown="\"Waiting for Stop\", \"Waiting for Stop (Acq Stopped)\"" w280 {
          selector: w280 -> [w284 _ _ _ _]
          tunnel: [w284 UI_State."Waiting for Exit (Acq Stopped)" ("UI State") UI_State."Waiting for Stop (Acq Stopped)" ("UI State") UI_State."Idle" ("UI State") UI_State."Idle" ("UI State")] -> w279
          tunnel: w278 -> [w283 w285 w287 w293 w299]
          tunnel: [w283 w285 w287 w292 w298] -> w277
          tunnel: w276 -> [_ _ _ w291 w297]
          frame Default {
          }
          frame "Waiting for Exit", "Waiting for Exit (Acq Stopped)" {
          }
          frame "Waiting for Stop", "Waiting for Stop (Acq Stopped)" {
          }
          frame "Waiting for Exit (Log Stopped)" {
            # "如果正在等待退出且记录已结束，“采集停止”消息表示应退出。"
            n90 = call-poly "Enqueue Message.vi"("Priority Message? (F)"=TRUE, "error in (no error)"=w293, "Message"="Exit", "Message Queue"=w291) -> ("error out"=w292:errorcluster)  [unwired: 6 in, 1 out]
          }
          frame "Waiting for Stop (Log Stopped)" {
            # "当前状态为等待停止时，如已停止记录，则收到\"Acquisition Stopped\"消息时即可停止。"
            n91 = call-poly "Enqueue Message.vi"("error in (no error)"=w299, "Message Data"="Ready..." ("Message"), "Message"="Update Status", "Message Queue"=w297) -> ("error out"=w298:errorcluster)  [unwired: 6 in, 1 out]
          }
        }
      }
      frame "Logging Stopped" {
        # "此处代码用于确定记录停止时采取何种操作。"
        n92 = case shown="\"Waiting for Stop (Acq Stopped)\"" w305 {
          selector: w305 -> [w309 _ _ _ _]
          tunnel: [w309 UI_State."Waiting for Exit (Log Stopped)" ("UI State") UI_State."Waiting for Stop (Log Stopped)" ("UI State") UI_State."Idle" ("UI State") UI_State."Idle" ("UI State")] -> w304
          tunnel: w303 -> [w308 w310 w312 w318 w324]
          tunnel: [w308 w310 w312 w317 w323] -> w302
          tunnel: w301 -> [_ _ _ w316 w322]
          frame Default {
          }
          frame "Waiting for Exit", "Waiting for Exit (Log Stopped)" {
          }
          frame "Waiting for Stop", "Waiting for Stop (Log Stopped)" {
          }
          frame "Waiting for Exit (Acq Stopped)" {
            # "如果正在等待退出且采集已结束，“记录停止”消息表示应退出。"
            n93 = call-poly "Enqueue Message.vi"("Priority Message? (F)"=TRUE, "error in (no error)"=w318, "Message"="Exit", "Message Queue"=w316) -> ("error out"=w317:errorcluster)  [unwired: 6 in, 1 out]
          }
          frame "Waiting for Stop (Acq Stopped)" {
            # "如果正在等待停止且采集已结束，“记录停止”消息表示应停止。"
            n94 = call-poly "Enqueue Message.vi"("error in (no error)"=w324, "Message Data"="Ready..." ("Message"), "Message"="Update Status", "Message Queue"=w322) -> ("error out"=w323:errorcluster)  [unwired: 6 in, 1 out]
          }
        }
      }
      frame "Broadcast settings" {
        w327 = "Update Settings" ("Message")
        # "向“记录和采集”消息队列发送“更新设置”消息。"
        n95 = Unbundle By Name(w341) -> ("Action Configuration"=w331:T7, "Hardware Configuration"=w340:T5, "Logging Configuration"=w339:T6, "所有测试项目任务"=w326:T18)
        n96 = call-poly "Enqueue Message.vi"("error in (no error)"=w333, "Message Data"=w331, "Message"=w327, "Message Queue"=w332) -> ("error out"=w334:errorcluster)  [unwired: 6 in, 1 out]
        n97 = call-poly "Enqueue Message.vi"("error in (no error)"=w334, "Message Data"=w340, "Message"=w327, "Message Queue"=w337) -> ("error out"=w342:errorcluster)  [unwired: 6 in, 1 out]
        n98 = call-poly "Enqueue Message.vi"("error in (no error)"=w342, "Message Data"=w339, "Message"=w327, "Message Queue"=w336) -> ("error out"=w330:errorcluster)  [unwired: 6 in, 1 out]
        n99 = call-poly "Enqueue Message.vi"("error in (no error)"=w330, "Message Data"=w326, "Message"=w327, "Message Queue"=w328) -> ("error out"=w329:errorcluster)  [unwired: 6 in, 1 out]
        n100 = Merge Errors(w329, w333) -> (w343:errorcluster)
      }
      frame "Launch Settings Dialog" {
        # "用户单击“设置”按钮时，启动设置对话框。"
        n101 = call "Settings Dialog.vi"("error in (no error)"=w351, "Settings in"=w352) -> ("error out"=w344:errorcluster, "Cancelled?"=w345:bool, "Settings out"=w349:T4)  [unwired: 6 in, 1 out]
        n102 = case shown="False" w345 {
          tunnel: w350 -> [w356 _]
          tunnel: w344 -> [w355 w357]
          tunnel: [w354 w357] -> w348
          frame False {
            n103 = call-poly "Enqueue Message.vi"("error in (no error)"=w355, "Message"="Broadcast Settings", "Message Queue"=w356) -> ("error out"=w354:errorcluster)  [unwired: 7 in, 1 out]
          }
          frame True {
          }
        }
      }
      frame "Error" {
        # "Error - 检查错误消息数据及其响应。该消息由应用程序各循环结束处的“错误处理”VI发送。"
        n104 = Variant To Data(error in=w363, type=errorcluster {"status"=FALSE, "code"=0, "source"=""} ("错误常量"), Variant=w362) -> (data=w360:errorcluster, error out=w359:errorcluster)
        n105 = call <vilib>:"Simple Error Handler.vi"("error in (no error)"=w359) -> ("error out"=w358:errorcluster)  [unwired: 4 in, 4 out]
        n106 = call <vilib>:"Simple Error Handler.vi"("error in (no error)"=w360) -> ("error out"=w364:errorcluster)  [unwired: 4 in, 4 out]
        n107 = call-poly "Enqueue Message.vi"("Priority Message? (F)"=TRUE, "Message"="Exit", "Message Queue"=w370) -> ("error out"=w367:errorcluster)  [unwired: 7 in, 1 out]
        n108 = Merge Errors(w367, w364, w358) -> (w366:errorcluster)
      }
      frame "Confirm Quit" {
        # "Confirm Quit - 该消息用于确认用户是否需要退出应用程序。"
        n109 = case shown="\"Acquiring and Logging\"" w377 {
          tunnel: w376 -> [w384 w390]
          tunnel: w375 -> [w383 w388]
          tunnel: [w380 w387] -> w374
          tunnel: [UI_State."Idle" ("UI State") w386] -> w373
          frame Default {
            # "如收到'Confirm Quit'消息时系统处于空闲状态，则不需要弹出确认提示。"
            n110 = call-poly "Enqueue Message.vi"("Priority Message? (F)"=TRUE, "error in (no error)"=w383, "Message"="Exit", "Message Queue"=w384) -> ("error out"=w380:errorcluster)  [unwired: 6 in, 1 out]
          }
          frame "Acquiring and Logging" {
            n111 = Two Button Dialog(message="采集仍在执行中，是否确定退出？" ("Confirm Quit Message"), 1:"否" ("No"), 2:"是" ("Yes")) -> (T button?=w389:bool)
            n112 = case shown="True" w389 {
              tunnel: w390 -> [_ w400]
              tunnel: w388 -> [w394 w399]
              tunnel: [w394 w398] -> w387
              tunnel: [UI_State."Acquiring and Logging" ("UI State") UI_State."Waiting for Exit" ("UI State")] -> w386
              frame False {
                # "用户不希望退出。"
              }
              frame True {
                n113 = call-poly "Enqueue Message.vi"("error in (no error)"=w399, "Message"="Stop", "Message Queue"=w400) -> ("error out"=w398:errorcluster)  [unwired: 7 in, 1 out]
              }
            }
          }
        }
      }
      frame "Exit" {
        w401 = TRUE ("Priority Message? (F)")
        w402 = "Exit" ("Message")
        # "不必检查错误输出。采集和记录队列可能已被释放。"
        # "停止VI。"
        # "Exit（退出）－触发用户事件，使“事件处理”循环停止运行。同时向“采集和记录”循环发送“退出”消息。"
        n114 = Release Queue(queue=w415, error in (no error)=w422) -> (error out=w413:errorcluster)  [unwired: 1 in, 2 out]
        n115 = call "Fire User Event - Stop.vi"("User Event - Stop"=w421) -> ("error out"=w420:errorcluster)  [unwired: 10 in]
        n116 = Release Notifier(notifier=w414, error in (no error)=w413) -> (error out=w412:errorcluster)  [unwired: 1 in, 2 out]
        n117 = Release Queue(queue=w411, error in (no error)=w412) -> (error out=w408:errorcluster)  [unwired: 1 in, 2 out]
        n118 = call-poly "Enqueue Message.vi"("Priority Message? (F)"=TRUE, "Message"=w402, "Message Queue"=w417) -> ()  [unwired: 7 in, 2 out]
        n119 = Release Queue(queue=w406, error in (no error)=w408) -> (error out=w407:errorcluster)  [unwired: 1 in, 2 out]
        n120 = call-poly "Enqueue Message.vi"("Priority Message? (F)"=w401, "Message"=w402, "Message Queue"=w416) -> ()  [unwired: 7 in, 2 out]
        n121 = call-poly "Enqueue Message.vi"("Priority Message? (F)"=w401, "Message"=w402, "Message Queue"=w405) -> ()  [unwired: 7 in, 2 out]
        n122 = call-poly "Enqueue Message.vi"("Priority Message? (F)"=w401, "Message"=w402, "Message Queue"=w404) -> ()  [unwired: 7 in, 2 out]
        n123 = call-poly "Enqueue Message.vi"("Priority Message? (F)"=w401, "Message"=w402, "Message Queue"=w403) -> ()  [unwired: 7 in, 2 out]
        n124 = Merge Errors(w420, w407) -> (w423:errorcluster)
      }
      frame "---Copy This Frame---" {
        # "如需创建新消息，可创建该帧的副本。在副本中，将本注释更改为对应消息的注释。"
        n125 = Merge Errors(w429) -> (w428:errorcluster)
      }
      frame "Update Write Log Settings" {
        # "如需创建新消息，可创建该帧的副本。在副本中，将本注释更改为对应消息的注释。"
        n126 = Variant To Data(error in=w436, type=T6 {"Log File Base Path"=path "", "电压传感器转换率"=[], "电压传感器本底"=[], "测试模式是否需要保存数据？"=FALSE} ("Logging Configuration"), Variant=w434) -> (data=w431:T6, error out=w433:errorcluster)
        n127 = Bundle By Name(cluster=w432, "Logging Configuration"=w431) -> (w430:T4)
        n128 = call "Get Config File Path.vi"("error in (no error)"=w433) -> ("error out"=w437:errorcluster, "XML File Path"=w440:path)  [unwired: 9 in]
        n129 = Flatten To XML(anything=w430) -> (xml string=w439:string)
        n130 = call-poly <vilib>:"Write to XML File.vi"("error in (no error)"=w437, "XML Input"=w439, "XML File Path"=w440) -> ("error out"=w438:errorcluster)  [unwired: 6 in, 2 out]
        n131 = Merge Errors(w438) -> (w443:errorcluster)
      }
      frame "Update Sensor Value" {
        # "如需创建新消息，可创建该帧的副本。在副本中，将本注释更改为对应消息的注释。"
        n132 = call-poly "Enqueue Message.vi"("error in (no error)"=w447, "Message Data"=w444, "Message"="Update Value", "Message Queue"=w445) -> ("error out"=w446:errorcluster)  [unwired: 6 in, 1 out]
        n133 = Merge Errors(w446) -> (w452:errorcluster)
      }
      frame "Move" {
        # "如需创建新消息，可创建该帧的副本。在副本中，将本注释更改为对应消息的注释。"
        n134 = Variant To Data(error in=w460, type=0.0, Variant=w459) -> (data=w454:dbl, error out=w457:errorcluster)
        n135 = call-poly "Enqueue Message.vi"("error in (no error)"=w457, "Message Data"=w454, "Message"="Move", "Message Queue"=w456) -> ("error out"=w453:errorcluster)  [unwired: 6 in, 1 out]
        n136 = Merge Errors(w453) -> (w464:errorcluster)
      }
      frame "啮合Start" {
        # "首先发送画曲线开始指令，然后发送内泄漏控制逻辑指令。"
        # "Start（开始） - 对于已经开始的采集，启用/禁用各个按钮并更新状态显示。"
        n137 = call-poly "Enqueue Message.vi"("error in (no error)"=w474, "Message Data"=Measure_Type."啮合" ("测试类型"), "Message"="画曲线开始", "Message Queue"=w475) -> ("error out"=w467:errorcluster)  [unwired: 6 in, 1 out]
        n138 = call-poly "Enqueue Message.vi"("error in (no error)"=w467, "Message"="啮合Start", "Message Queue"=w468) -> ("error out"=w469:errorcluster)  [unwired: 7 in, 1 out]
        n139 = Merge Errors(w469) -> (w476:errorcluster)
      }
      frame "退回Start" {
        # "首先发送画曲线开始指令，然后发送内泄漏控制逻辑指令。"
        # "Start（开始） - 对于已经开始的采集，启用/禁用各个按钮并更新状态显示。"
        n140 = call-poly "Enqueue Message.vi"("error in (no error)"=w486, "Message Data"=Measure_Type."退回" ("测试类型"), "Message"="画曲线开始", "Message Queue"=w487) -> ("error out"=w479:errorcluster)  [unwired: 6 in, 1 out]
        n141 = call-poly "Enqueue Message.vi"("error in (no error)"=w479, "Message"="自动调阀测试_内泄漏Start", "Message Queue"=w480) -> ("error out"=w481:errorcluster)  [unwired: 7 in, 1 out]
        n142 = Merge Errors(w481) -> (w488:errorcluster)
      }
      frame "功能Start" {
        # "首先发送画曲线开始指令，然后发送内泄漏控制逻辑指令。"
        # "Start（开始） - 对于已经开始的采集，启用/禁用各个按钮并更新状态显示。"
        n143 = call-poly "Enqueue Message.vi"("error in (no error)"=w498, "Message Data"=Measure_Type."功能" ("测试类型"), "Message"="画曲线开始", "Message Queue"=w499) -> ("error out"=w491:errorcluster)  [unwired: 6 in, 1 out]
        n144 = call-poly "Enqueue Message.vi"("error in (no error)"=w491, "Message"="自动调阀测试_内泄漏Start", "Message Queue"=w492) -> ("error out"=w493:errorcluster)  [unwired: 7 in, 1 out]
        n145 = Merge Errors(w493) -> (w500:errorcluster)
      }
      frame "力特性Start" {
        # "首先发送画曲线开始指令，然后发送内泄漏控制逻辑指令。"
        # "Start（开始） - 对于已经开始的采集，启用/禁用各个按钮并更新状态显示。"
        n146 = call-poly "Enqueue Message.vi"("error in (no error)"=w510, "Message Data"=Measure_Type."力特性" ("测试类型"), "Message"="画曲线开始", "Message Queue"=w511) -> ("error out"=w503:errorcluster)  [unwired: 6 in, 1 out]
        n147 = call-poly "Enqueue Message.vi"("error in (no error)"=w503, "Message"="自动调阀测试_内泄漏Start", "Message Queue"=w504) -> ("error out"=w505:errorcluster)  [unwired: 7 in, 1 out]
        n148 = Merge Errors(w505) -> (w512:errorcluster)
      }
      frame "DAQ Reset" {
        # "如需创建新消息，可创建该帧的副本。在副本中，将本注释更改为对应消息的注释。"
        n149 = Unbundle By Name(w514) -> ("Hardware Configuration.电压读取设置.device in"=w513:tag)
        n150 = call <vilib>:"DAQmx Reset Device.vi"("device in"=w513, "error in"=w516) -> ("error out"=w515:errorcluster)  [unwired: 13 in]
        n151 = Merge Errors(w515) -> (w519:errorcluster)
      }
      frame "Clear" {
        # "通知采集线程采集一次，通知log线程计算一个转换值，等待log线程计算转换完之后，\nplot线程通知UI线程，更新数据。"
        n152 = call-poly "Enqueue Message.vi"("error in (no error)"=w526, "Message"="Acquire Once", "Message Queue"=w525) -> ("error out"=w523:errorcluster)  [unwired: 7 in, 1 out]
        n153 = call-poly "Enqueue Message.vi"("error in (no error)"=w523, "Message"="Clear Zero", "Message Queue"=w522) -> ("error out"=w520:errorcluster)  [unwired: 7 in, 1 out]
        n154 = Merge Errors(w520) -> (w530:errorcluster)
      }
      frame "Clear Old" {
        # "通知Acquire线程采集一次，然后log线程更新本底。"
        n155 = call "Acquire Once.vi"("error in (no error)"=w540, "Settings"=w534) -> ("error out"=w539:errorcluster, "信号数据"=w532:dbl[][])  [unwired: 7 in, 1 out]
        n156 = for {
          tunnel: w532 -> [w545] mode=indexing
          tunnel: [w544] -> w531 mode=indexing
          n157 = call-poly <vilib>:"Mean.vi"("X"=w545) -> ("mean"=w544:dbl)  [unwired: 1 out]
        }
        n158 = Bundle By Name(cluster=w534, "Logging Configuration.电压传感器本底"=w531) -> (w533:T4)
        n159 = call "Save Settings to XML.vi"("error in (no error)"=w539, "Settings"=w533) -> ("error out"=w536:errorcluster)  [unwired: 9 in]
        n160 = call-poly "Enqueue Message.vi"("error in (no error)"=w536, "Message"="Broadcast Settings", "Message Queue"=w537) -> ("error out"=w535:errorcluster)  [unwired: 7 in, 1 out]
        n161 = Merge Errors(w535) -> (w543:errorcluster)
      }
      frame "Read" {
        # "通知采集线程采集一次，通知log线程计算一个转换值，等待log线程计算转换完之后，\nplot线程通知UI线程，更新数据。"
        n162 = call-poly "Enqueue Message.vi"("error in (no error)"=w552, "Message"="Acquire Once", "Message Queue"=w551) -> ("error out"=w549:errorcluster)  [unwired: 7 in, 1 out]
        n163 = call-poly "Enqueue Message.vi"("error in (no error)"=w549, "Message"="Compute No Log", "Message Queue"=w548) -> ("error out"=w546:errorcluster)  [unwired: 7 in, 1 out]
        n164 = Merge Errors(w546) -> (w556:errorcluster)
      }
      frame "Read Old" {
        # "如需创建新消息，可创建该帧的副本。在副本中，将本注释更改为对应消息的注释。"
        n165 = call "Acquire Once.vi"("error in (no error)"=w566, "Settings"=w564) -> ("error out"=w561:errorcluster, "信号数据"=w565:dbl[][])  [unwired: 7 in, 1 out]
        n166 = Unbundle By Name(w564) -> ("Logging Configuration.电压传感器转换率"=w563:dbl[], "Logging Configuration.电压传感器本底"=w562:dbl[])
        n167 = call "GetDatas.vi"("电压传感器本地"=w562, "电压传感器转换率"=w563, "信号数据"=w565) -> ("传感器信号"=w557:dbl[])  [unwired: 8 in]
        n168 = call-poly "Enqueue Message.vi"("error in (no error)"=w561, "Message Data"=w557, "Message"="Update Value", "Message Queue"=w559) -> ("error out"=w560:errorcluster)  [unwired: 6 in, 1 out]
        n169 = Merge Errors(w560) -> (w569:errorcluster)
      }
      frame "Calculate" {
        # "发指令让记录线程执行计算，传入相应的计算类型。"
        # "如需创建新消息，可创建该帧的副本。在副本中，将本注释更改为对应消息的注释。"
        n170 = Variant To Data(error in=w574, type=Measure_Type."啮合" ("计算类型"), Variant=w572) -> (data=w570:T21, error out=w573:errorcluster)
        n171 = call-poly "Enqueue Message.vi"("error in (no error)"=w573, "Message Data"=w570, "Message"="Calculate", "Message Queue"=w576) -> ("error out"=w577:errorcluster)  [unwired: 6 in, 1 out]
        n172 = Merge Errors(w577) -> (w581:errorcluster)
      }
      frame "Log Once" {
        # "发指令让记录线程执行计算，传入相应的计算类型。"
        # "如需创建新消息，可创建该帧的副本。在副本中，将本注释更改为对应消息的注释。"
        n173 = call-poly "Enqueue Message.vi"("error in (no error)"=w585, "Message"="Log Once", "Message Queue"=w582) -> ("error out"=w584:errorcluster)  [unwired: 7 in, 1 out]
        n174 = Merge Errors(w584) -> (w589:errorcluster)
      }
      frame "等待开始按钮" {
        # "如需创建新消息，可创建该帧的副本。在副本中，将本注释更改为对应消息的注释。"
        n175 = call-poly "Enqueue Message.vi"("error in (no error)"=w594, "Message Data"=w590, "Message"="自动调阀测试 等待开始按钮", "Message Queue"=w592) -> ("error out"=w593:errorcluster)  [unwired: 6 in, 1 out]
        n176 = Merge Errors(w593) -> (w598:errorcluster)
      }
      frame "夹紧/松阀总" {
        # "如需创建新消息，可创建该帧的副本。在副本中，将本注释更改为对应消息的注释。"
        n177 = call-poly "Enqueue Message.vi"("error in (no error)"=w603, "Message Data"=w599, "Message"="自动调阀测试 夹紧/松阀总", "Message Queue"=w601) -> ("error out"=w602:errorcluster)  [unwired: 6 in, 1 out]
        n178 = Merge Errors(w602) -> (w607:errorcluster)
      }
      frame "夹紧/松阀芯" {
        # "如需创建新消息，可创建该帧的副本。在副本中，将本注释更改为对应消息的注释。"
        n179 = call-poly "Enqueue Message.vi"("error in (no error)"=w612, "Message Data"=w608, "Message"="自动调阀测试 夹紧/松阀芯", "Message Queue"=w610) -> ("error out"=w611:errorcluster)  [unwired: 6 in, 1 out]
        n180 = Merge Errors(w611) -> (w616:errorcluster)
      }
      frame "内泄漏开始" {
        # "首先发送画曲线开始指令，然后发送内泄漏控制逻辑指令。"
        # "Start（开始） - 对于已经开始的采集，启用/禁用各个按钮并更新状态显示。"
        n181 = call-poly "Enqueue Message.vi"("error in (no error)"=w619, "Message"="clear", "Message Queue"=w621) -> ("error out"=w618:errorcluster, "dup Message Queue"=w620:refnum<queue>)  [unwired: 7 in]
        n182 = call-poly "Enqueue Message.vi"("error in (no error)"=w618, "Message Data"=Measure_Type."内泄漏" ("测试类型"), "Message"="画曲线开始", "Message Queue"=w620) -> ("error out"=w624:errorcluster)  [unwired: 6 in, 1 out]
        n183 = call-poly "Enqueue Message.vi"("error in (no error)"=w624, "Message"="自动调阀测试_内泄漏Start", "Message Queue"=w625) -> ("error out"=w626:errorcluster)  [unwired: 7 in, 1 out]
        n184 = Merge Errors(w626) -> (w631:errorcluster)
      }
      frame "电机使能" {
        # "如需创建新消息，可创建该帧的副本。在副本中，将本注释更改为对应消息的注释。"
        n185 = call-poly "Enqueue Message.vi"("error in (no error)"=w636, "Message Data"=w632, "Message"="自动调阀测试 电机使能", "Message Queue"=w634) -> ("error out"=w635:errorcluster)  [unwired: 6 in, 1 out]
        n186 = Merge Errors(w635) -> (w640:errorcluster)
      }
      frame "内泄漏开/停" {
        # "如需创建新消息，可创建该帧的副本。在副本中，将本注释更改为对应消息的注释。"
        n187 = call-poly "Enqueue Message.vi"("error in (no error)"=w645, "Message Data"=w641, "Message"="自动调阀测试 内泄漏开/停", "Message Queue"=w643) -> ("error out"=w644:errorcluster)  [unwired: 6 in, 1 out]
        n188 = Merge Errors(w644) -> (w649:errorcluster)
      }
      frame "内泄漏停" {
        # "如需创建新消息，可创建该帧的副本。在副本中，将本注释更改为对应消息的注释。"
        n189 = call-poly "Enqueue Message.vi"("error in (no error)"=w653, "Message"="自动调阀测试 内泄漏停", "Message Queue"=w651) -> ("error out"=w652:errorcluster)  [unwired: 7 in, 1 out]
        n190 = Merge Errors(w652) -> (w657:errorcluster)
      }
      frame "内泄漏放油" {
        # "如需创建新消息，可创建该帧的副本。在副本中，将本注释更改为对应消息的注释。"
        n191 = call-poly "Enqueue Message.vi"("error in (no error)"=w662, "Message Data"=w658, "Message"="自动调阀测试 内泄漏放油", "Message Queue"=w660) -> ("error out"=w661:errorcluster)  [unwired: 6 in, 1 out]
        n192 = Merge Errors(w661) -> (w666:errorcluster)
      }
      frame "方向机供油" {
        # "如需创建新消息，可创建该帧的副本。在副本中，将本注释更改为对应消息的注释。"
        n193 = call-poly "Enqueue Message.vi"("error in (no error)"=w671, "Message Data"=w667, "Message"="自动调阀测试 方向机供油", "Message Queue"=w669) -> ("error out"=w670:errorcluster)  [unwired: 6 in, 1 out]
        n194 = Merge Errors(w670) -> (w675:errorcluster)
      }
      frame "分中Start" {
        # "首先发送画曲线开始指令，然后发送内泄漏控制逻辑指令。"
        # "Start（开始） - 对于已经开始的采集，启用/禁用各个按钮并更新状态显示。"
        n195 = call-poly "Enqueue Message.vi"("error in (no error)"=w685, "Message Data"=Measure_Type."分中" ("测试类型"), "Message"="画曲线开始", "Message Queue"=w686) -> ("error out"=w678:errorcluster)  [unwired: 6 in, 1 out]
        n196 = call-poly "Enqueue Message.vi"("error in (no error)"=w678, "Message"="自动调阀测试_分中Start", "Message Queue"=w679) -> ("error out"=w680:errorcluster)  [unwired: 7 in, 1 out]
        n197 = Merge Errors(w680) -> (w687:errorcluster)
      }
      frame "分中_更新停止角度" {
        # "向“记录和采集”消息队列发送“更新设置”消息。"
        n198 = Variant To Data(error in=w694, type=0.0, Variant=w693) -> (data=w689:dbl, error out=w691:errorcluster)
        n199 = call-poly "Enqueue Message.vi"("error in (no error)"=w691, "Message Data"=w689, "Message"="自动调阀测试_分中更新停止角度", "Message Queue"=w696) -> ("error out"=w695:errorcluster)  [unwired: 6 in, 1 out]
        n200 = Merge Errors(w695) -> (w699:errorcluster)
      }
      frame "分中Calculate" {
        # "向“记录和采集”消息队列发送“更新设置”消息。"
        n201 = call-poly "Enqueue Message.vi"("error in (no error)"=w700, "Message"="Calculate分中", "Message Queue"=w701) -> ("error out"=w703:errorcluster)  [unwired: 7 in, 1 out]
        n202 = Merge Errors(w703) -> (w707:errorcluster)
      }
      frame "对中Start" {
        # "首先发送画曲线开始指令，然后发送内泄漏控制逻辑指令。"
        # "Start（开始） - 对于已经开始的采集，启用/禁用各个按钮并更新状态显示。"
        n203 = call-poly "Enqueue Message.vi"("error in (no error)"=w710, "Message"="clear", "Message Queue"=w712) -> ("error out"=w709:errorcluster, "dup Message Queue"=w711:refnum<queue>)  [unwired: 7 in]
        n204 = call-poly "Enqueue Message.vi"("error in (no error)"=w709, "Message Data"=Measure_Type."对中" ("测试类型"), "Message"="画曲线开始", "Message Queue"=w711) -> ("error out"=w715:errorcluster)  [unwired: 6 in, 1 out]
        n205 = call-poly "Enqueue Message.vi"("error in (no error)"=w715, "Message"="自动调阀测试_对中Start", "Message Queue"=w716) -> ("error out"=w717:errorcluster)  [unwired: 7 in, 1 out]
        n206 = Merge Errors(w717) -> (w722:errorcluster)
      }
      frame "对中计算" {
        # "如需创建新消息，可创建该帧的副本。在副本中，将本注释更改为对应消息的注释。"
        n207 = call-poly "Enqueue Message.vi"("error in (no error)"=w727, "Message Data"=Measure_Type."对中" ("计算类型"), "Message"="Calculate", "Message Queue"=w723) -> ("error out"=w726:errorcluster)  [unwired: 6 in, 1 out]
        n208 = Merge Errors(w726) -> (w731:errorcluster)
      }
      frame "对中Calculate" {
        # "如需创建新消息，可创建该帧的副本。在副本中，将本注释更改为对应消息的注释。"
        n209 = call-poly "Enqueue Message.vi"("error in (no error)"=w735, "Message"="Calculate对中", "Message Queue"=w732) -> ("error out"=w734:errorcluster)  [unwired: 7 in, 1 out]
        n210 = Merge Errors(w734) -> (w739:errorcluster)
      }
      frame "自动对中Move" {
        w746 = "自动调阀测试 卡盘松/紧" ("Message")
        w768 = "自动调阀测试 电机使能" ("Message")
        w741 = "Wait" ("Message")
        w777 = "自动调阀测试 扭杆紧/松" ("Message")
        # "自动调阀测试 扭杆紧/松"
        # "如需创建新消息，可创建该帧的副本。在副本中，将本注释更改为对应消息的注释。"
        n211 = Variant To Data(error in=w790, type=0.0, Variant=w789) -> (data=w753:dbl, error out=w784:errorcluster)
        n212 = call-poly "Enqueue Message.vi"("error in (no error)"=w784, "Message Data"=FALSE, "Message"=w777, "Message Queue"=w785) -> ("error out"=w782:errorcluster, "dup Message Queue"=w781:refnum<queue>)  [unwired: 6 in]
        n213 = call-poly "Enqueue Message.vi"("error in (no error)"=w782, "Message Data"=2.0, "Message"=w741, "Message Queue"=w781) -> ("error out"=w779:errorcluster, "dup Message Queue"=w778:refnum<queue>)  [unwired: 6 in]
        n214 = call-poly "Enqueue Message.vi"("error in (no error)"=w779, "Message Data"=TRUE, "Message"=w777, "Message Queue"=w778) -> ("error out"=w774:errorcluster, "dup Message Queue"=w775:refnum<queue>)  [unwired: 6 in]
        n215 = call-poly "Enqueue Message.vi"("error in (no error)"=w774, "Message Data"=2.0, "Message"=w741, "Message Queue"=w775) -> ("error out"=w772:errorcluster, "dup Message Queue"=w771:refnum<queue>)  [unwired: 6 in]
        n216 = call-poly "Enqueue Message.vi"("error in (no error)"=w772, "Message Data"=FALSE, "Message"=w768, "Message Queue"=w771) -> ("error out"=w766:errorcluster, "dup Message Queue"=w765:refnum<queue>)  [unwired: 6 in]
        n217 = call-poly "Enqueue Message.vi"("error in (no error)"=w766, "Message Data"=2.0, "Message"=w741, "Message Queue"=w765) -> ("error out"=w763:errorcluster, "dup Message Queue"=w764:refnum<queue>)  [unwired: 6 in]
        n218 = call-poly "Enqueue Message.vi"("error in (no error)"=w763, "Message Data"=FALSE, "Message"=w746, "Message Queue"=w764) -> ("error out"=w761:errorcluster, "dup Message Queue"=w759:refnum<queue>)  [unwired: 6 in]
        n219 = call-poly "Enqueue Message.vi"("error in (no error)"=w761, "Message Data"=2.0, "Message"=w741, "Message Queue"=w759) -> ("error out"=w760:errorcluster, "dup Message Queue"=w758:refnum<queue>)  [unwired: 6 in]
        n220 = call-poly "Enqueue Message.vi"("error in (no error)"=w760, "Message Data"=TRUE, "Message"=w768, "Message Queue"=w758) -> ("error out"=w755:errorcluster, "dup Message Queue"=w756:refnum<queue>)  [unwired: 6 in]
        n221 = call-poly "Enqueue Message.vi"("error in (no error)"=w755, "Message Data"=w753, "Message"="Move", "Message Queue"=w756) -> ("error out"=w750:errorcluster, "dup Message Queue"=w751:refnum<queue>)  [unwired: 6 in]
        n222 = call-poly "Enqueue Message.vi"("error in (no error)"=w750, "Message Data"=2.0, "Message"=w741, "Message Queue"=w751) -> ("error out"=w747:errorcluster, "dup Message Queue"=w748:refnum<queue>)  [unwired: 6 in]
        n223 = call-poly "Enqueue Message.vi"("error in (no error)"=w747, "Message Data"=FALSE, "Message"=w746, "Message Queue"=w748) -> ("error out"=w743:errorcluster, "dup Message Queue"=w744:refnum<queue>)  [unwired: 6 in]
        n224 = call-poly "Enqueue Message.vi"("error in (no error)"=w743, "Message Data"=2.0, "Message"=w741, "Message Queue"=w744) -> ("error out"=w742:errorcluster)  [unwired: 6 in, 1 out]
        n225 = call-poly "Enqueue Message.vi"("error in (no error)"=w742, "Message"="自动调阀测试 自动对中", "Message Queue"=w740) -> ("error out"=w786:errorcluster)  [unwired: 7 in, 1 out]
        n226 = Merge Errors(w786) -> (w794:errorcluster)
      }
      frame "自动对中完成" {
        # "如需创建新消息，可创建该帧的副本。在副本中，将本注释更改为对应消息的注释。"
        n227 = call-poly "Enqueue Message.vi"("error in (no error)"=w799, "Message Data"="对中" ("Message"), "Message"="Update Finish Task", "Message Queue"=w797) -> ("error out"=w798:errorcluster)  [unwired: 6 in, 1 out]
        n228 = call-poly "Enqueue Message.vi"("error in (no error)"=w798, "Message"="完成", "Message Queue"=w800) -> ("error out"=w802:errorcluster)  [unwired: 7 in, 1 out]
        n229 = Merge Errors(w802) -> (w806:errorcluster)
      }
      frame "扭杆紧/松" {
        # "如需创建新消息，可创建该帧的副本。在副本中，将本注释更改为对应消息的注释。"
        n230 = call-poly "Enqueue Message.vi"("error in (no error)"=w811, "Message Data"=w807, "Message"="自动调阀测试 扭杆紧/松", "Message Queue"=w809) -> ("error out"=w810:errorcluster)  [unwired: 6 in, 1 out]
        n231 = Merge Errors(w810) -> (w815:errorcluster)
      }
      frame "托起油缸上/下" {
        # "如需创建新消息，可创建该帧的副本。在副本中，将本注释更改为对应消息的注释。"
        n232 = call-poly "Enqueue Message.vi"("error in (no error)"=w819, "Message"="自动调阀测试 托起油缸上/下", "Message Queue"=w817) -> ("error out"=w818:errorcluster)  [unwired: 7 in, 1 out]
        n233 = Merge Errors(w818) -> (w823:errorcluster)
      }
      frame "卡盘松/紧" {
        # "如需创建新消息，可创建该帧的副本。在副本中，将本注释更改为对应消息的注释。"
        n234 = call-poly "Enqueue Message.vi"("error in (no error)"=w828, "Message Data"=w824, "Message"="自动调阀测试 卡盘松/紧", "Message Queue"=w826) -> ("error out"=w827:errorcluster)  [unwired: 6 in, 1 out]
        n235 = Merge Errors(w827) -> (w832:errorcluster)
      }
      frame "数控启动钻孔" {
        # "如需创建新消息，可创建该帧的副本。在副本中，将本注释更改为对应消息的注释。"
        n236 = call-poly "Enqueue Message.vi"("error in (no error)"=w836, "Message"="自动调阀测试 数控启动钻孔", "Message Queue"=w834) -> ("error out"=w835:errorcluster)  [unwired: 7 in, 1 out]
        n237 = Merge Errors(w835) -> (w840:errorcluster)
      }
      frame "全自动调阀测试" {
        # "如需创建新消息，可创建该帧的副本。在副本中，将本注释更改为对应消息的注释。"
        n238 = call-poly "Enqueue Message.vi"("error in (no error)"=w844, "Message"="全自动调阀测试", "Message Queue"=w842) -> ("error out"=w843:errorcluster)  [unwired: 7 in, 1 out]
        n239 = Merge Errors(w843) -> (w848:errorcluster)
      }
      frame "自动调阀测试 夹紧阀总" {
        # "如需创建新消息，可创建该帧的副本。在副本中，将本注释更改为对应消息的注释。"
        n240 = call-poly "Enqueue Message.vi"("error in (no error)"=w853, "Message Data"=TRUE, "Message"="自动调阀测试 夹紧/松阀总", "Message Queue"=w850) -> ("error out"=w852:errorcluster)  [unwired: 6 in, 1 out]
        n241 = Merge Errors(w852) -> (w857:errorcluster)
      }
      frame "自动调阀测试 夹紧阀芯" {
        # "如需创建新消息，可创建该帧的副本。在副本中，将本注释更改为对应消息的注释。"
        n242 = call-poly "Enqueue Message.vi"("error in (no error)"=w862, "Message Data"=TRUE, "Message"="自动调阀测试 夹紧/松阀芯", "Message Queue"=w859) -> ("error out"=w861:errorcluster)  [unwired: 6 in, 1 out]
        n243 = Merge Errors(w861) -> (w866:errorcluster)
      }
      frame "自动调阀测试 电机使能" {
        # "如需创建新消息，可创建该帧的副本。在副本中，将本注释更改为对应消息的注释。"
        n244 = call-poly "Enqueue Message.vi"("error in (no error)"=w871, "Message Data"=TRUE, "Message"="自动调阀测试 电机使能", "Message Queue"=w868) -> ("error out"=w870:errorcluster)  [unwired: 6 in, 1 out]
        n245 = Merge Errors(w870) -> (w875:errorcluster)
      }
      frame "自动调阀测试 内泄漏开始" {
        # "首先发送画曲线开始指令，然后发送内泄漏控制逻辑指令。"
        # "Start（开始） - 对于已经开始的采集，启用/禁用各个按钮并更新状态显示。"
        n246 = call-poly "Enqueue Message.vi"("error in (no error)"=w878, "Message"="clear", "Message Queue"=w880) -> ("error out"=w877:errorcluster, "dup Message Queue"=w879:refnum<queue>)  [unwired: 7 in]
        n247 = call-poly "Enqueue Message.vi"("error in (no error)"=w877, "Message Data"=Measure_Type."内泄漏" ("测试类型"), "Message"="画曲线开始", "Message Queue"=w879) -> ("error out"=w883:errorcluster)  [unwired: 6 in, 1 out]
        n248 = call-poly "Enqueue Message.vi"("error in (no error)"=w883, "Message"="自动调阀测试_内泄漏Start", "Message Queue"=w884) -> ("error out"=w885:errorcluster)  [unwired: 7 in, 1 out]
        n249 = Merge Errors(w885) -> (w890:errorcluster)
      }
      frame "自动调阀测试 自动分中" {
        # "首先发送画曲线开始指令，然后发送内泄漏控制逻辑指令。"
        # "Start（开始） - 对于已经开始的采集，启用/禁用各个按钮并更新状态显示。"
        n250 = call-poly "Enqueue Message.vi"("error in (no error)"=w900, "Message Data"=Measure_Type."分中" ("测试类型"), "Message"="画曲线开始", "Message Queue"=w901) -> ("error out"=w893:errorcluster)  [unwired: 6 in, 1 out]
        n251 = call-poly "Enqueue Message.vi"("error in (no error)"=w893, "Message"="自动调阀测试_自动分中Start", "Message Queue"=w894) -> ("error out"=w895:errorcluster)  [unwired: 7 in, 1 out]
        n252 = Merge Errors(w895) -> (w902:errorcluster)
      }
      frame "自动调阀测试 方向机供油" {
        # "如需创建新消息，可创建该帧的副本。在副本中，将本注释更改为对应消息的注释。"
        n253 = call-poly "Enqueue Message.vi"("error in (no error)"=w907, "Message Data"=TRUE, "Message"="自动调阀测试 方向机供油", "Message Queue"=w904) -> ("error out"=w906:errorcluster)  [unwired: 6 in, 1 out]
        n254 = Merge Errors(w906) -> (w911:errorcluster)
      }
      frame "自动调阀测试 扭杆紧" {
        # "如需创建新消息，可创建该帧的副本。在副本中，将本注释更改为对应消息的注释。"
        n255 = call-poly "Enqueue Message.vi"("error in (no error)"=w916, "Message Data"=TRUE, "Message"="自动调阀测试 扭杆紧/松", "Message Queue"=w913) -> ("error out"=w915:errorcluster)  [unwired: 6 in, 1 out]
        n256 = Merge Errors(w915) -> (w920:errorcluster)
      }
      frame "自动调阀测试 卡盘紧" {
        # "如需创建新消息，可创建该帧的副本。在副本中，将本注释更改为对应消息的注释。"
        n257 = call-poly "Enqueue Message.vi"("error in (no error)"=w925, "Message Data"=TRUE, "Message"="自动调阀测试 卡盘松/紧", "Message Queue"=w922) -> ("error out"=w924:errorcluster)  [unwired: 6 in, 1 out]
        n258 = Merge Errors(w924) -> (w929:errorcluster)
      }
      frame "自动调阀测试 自动对中" {
        # "首先发送画曲线开始指令，然后发送内泄漏控制逻辑指令。"
        # "Start（开始） - 对于已经开始的采集，启用/禁用各个按钮并更新状态显示。"
        n259 = call-poly "Enqueue Message.vi"("error in (no error)"=w932, "Message"="clear", "Message Queue"=w934) -> ("error out"=w931:errorcluster, "dup Message Queue"=w933:refnum<queue>)  [unwired: 7 in]
        n260 = call-poly "Enqueue Message.vi"("error in (no error)"=w931, "Message Data"=Measure_Type."对中" ("测试类型"), "Message"="画曲线开始", "Message Queue"=w933) -> ("error out"=w937:errorcluster)  [unwired: 6 in, 1 out]
        n261 = call-poly "Enqueue Message.vi"("error in (no error)"=w937, "Message"="自动调阀测试_自动对中Start", "Message Queue"=w938) -> ("error out"=w939:errorcluster)  [unwired: 7 in, 1 out]
        n262 = Merge Errors(w939) -> (w944:errorcluster)
      }
      frame Default {
        # "如得到的消息未经任何分支定义，则运行“默认”分支。输出程序错误。"
        n263 = xnode "错误下拉列表"("parameter 0"=w946) -> ("error out"=w947:errorcluster)
      }
    }
    n264 = call "Error Handler - Message Handling Loop.vi"("error in (no error)"=w25, "Message Queue"=w23) -> ("dup error in"=w24:errorcluster)  [unwired: 8 in, 1 out]
  }
  "error out" <- w4
